vi "User Access Level FGV Unit Test.vi"() -> ()   [LabVIEW 2014]
panel:
  in  "Access Secure Area":bool
  out "Error Out":errorcluster
  in  "Error In":errorcluster
  in  "Current User":string
  in  "Set User Access Level":bool
  in  "stop":bool
  # "1.  Set access level for current user."
  # "2.  Test access level by verifying the appropriate dialog message."
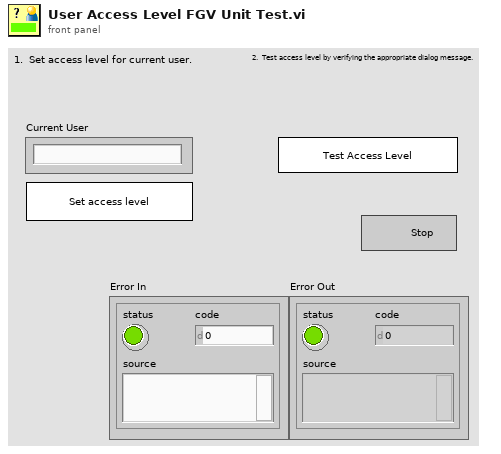
[diagram p1: front panel]
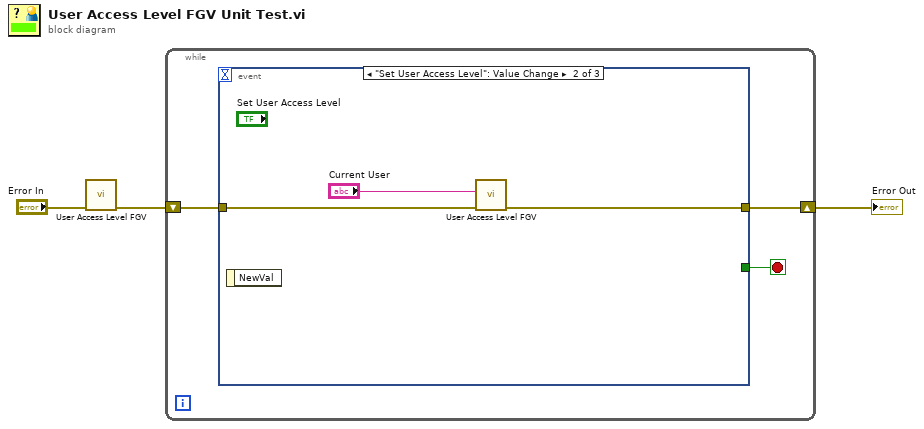
[diagram p0: block diagram]
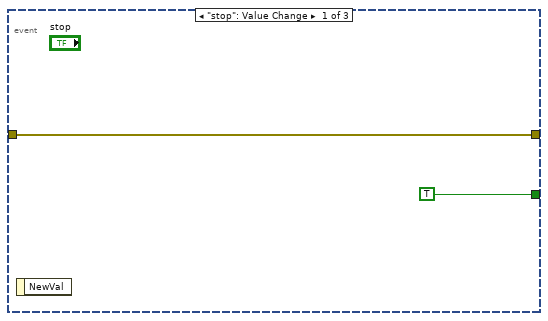
[diagram p2: hidden frame]
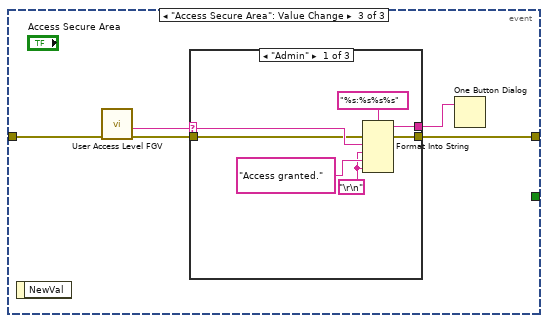
[diagram p3: hidden frame]
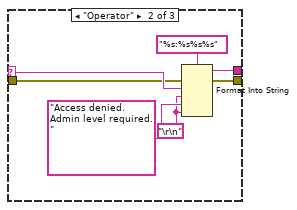
[diagram p4: hidden frame]
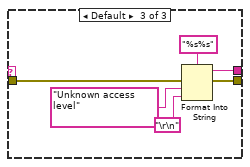
[diagram p5: hidden frame]
diagram:
  n1 = call "User Access Level FGV.vi"("Error In"="Error In") -> ("Error Out"=w3:errorcluster)  [unwired: 9 in, 1 out]
  n2 = while {
    shift-right: [w4] -> w1
    shift-left: w3 -> [w5]
    stop <- w6 stop-if-true
    n3 = event shown="[1] \"Set User Access Level\": Value Change" {
      selector: _ -> [_ _ _]
      dyn-events: _ -> [_ _ _]
      timeout: _ -> [_ _ _]
      tunnel: [TRUE ("stop") _ _] -> w6
      tunnel: w5 -> [w7 w11 w16]
      tunnel: [w7 w9 w15] -> w4
      event "stop": Value Change {
        n4 = event-data() -> ()  [unwired: 1 in, 1 out]
      }
      event "Set User Access Level": Value Change {
        n5 = event-data() -> ()  [unwired: 1 in, 1 out]
        n6 = call "User Access Level FGV.vi"("Error In"=w11, "User Name"="Current User") -> ("Error Out"=w9:errorcluster)  [unwired: 8 in, 1 out]
      }
      event "Access Secure Area": Value Change {
        n7 = event-data() -> ()  [unwired: 1 in, 1 out]
        n8 = call "User Access Level FGV.vi"("Error In"=w16) -> ("Error Out"=w14:errorcluster, "User Level"=w13:string)  [unwired: 9 in]
        n9 = case shown="\"Admin\"" w13 {
          selector: w13 -> [w23 w30 _]
          tunnel: [w21 w28 w35] -> w15
          tunnel: w14 -> [w22 w29 w36]
          tunnel: [w17 w24 w33] -> w12
          frame "Admin" {
            w19 = "\r\n"
            n10 = Format Into String(format string="%s:%s%s%s", error in=w22, w23, w19, "Access granted." ("message"), w19) -> (resulting string=w17:string, error out=w21:errorcluster)  [unwired: 1 in]
          }
          frame "Operator" {
            w26 = "\r\n"
            n11 = Format Into String(format string="%s:%s%s%s", error in=w29, w30, w26, "Access denied.  Admin level required." ("message"), w26) -> (resulting string=w24:string, error out=w28:errorcluster)  [unwired: 1 in]
          }
          frame Default {
            n12 = Format Into String(format string="%s%s", error in=w36, "Unknown access level" ("message"), "\r\n") -> (resulting string=w33:string, error out=w35:errorcluster)  [unwired: 1 in]
          }
        }
        n13 = One Button Dialog(message=w12) -> ()  [unwired: 1 in, 1 out]
      }
    }
  }
  "Error Out" <- w1
